vi "VNA_const_generator_spa.vi"() -> ()   [LabVIEW 2013]
panel:
  in  "?":enum32{"VNA (constant signal)"}(tab)
  in  "Power (dBm)":dbl caption="Center Freq (Hz):" min=1.0 max=19.0 format="%#.6p"
  in  "Frequency  (Hz)":dbl=20.0 caption="Center Freq (Hz):" min=1.0 max=20.0 format="%#.6p"
  in  "?":enum32{"RS generator with internal  modulation"}(tab)
  in  "Power start (dBm)":dbl=-50.0 caption="Center Freq (Hz):" min=1.0 max=20.0 format="%#.6p"
  in  "Frequency start (Hz)":dbl=2.0 caption="Center Freq (Hz):" min=1.0 max=19.0 format="%#.6p"
  in  "Power end (dBm)":dbl caption="Center Freq (Hz):" min=1.0 max=19.0 format="%#.6p"
  in  "Frequency end (Hz)":dbl=20.0 caption="Center Freq (Hz):" min=1.0 max=20.0 format="%#.6p"
  in  "power_points":i32=20 caption="Power N of points"
  in  "freq_points":i32=201 caption="Frequency N of points"
  in  "MOD frequency end  (Hz)":dbl=20.0 caption="Center Freq (Hz):" min=1.0 max=20.0 format="%#.6p"
  in  "MOD frequency start  (Hz)":dbl=20.0 caption="Center Freq (Hz):" min=1.0 max=20.0 format="%#.6p"
  in  "modulation_points":i32=20 caption="modulation N of points"
  in  "?":enum32{"SPA"}(tab)
  in  "Center freq (Hz)":dbl=-10.0 caption="Center Freq (Hz):" format="%#.6p"
  in  "Span (Hz)":dbl=-10.0 caption="Center Freq (Hz):" format="%#.6p"
  in  "RBW  (Hz)":dbl=-10.0 caption="Center Freq (Hz):" format="%#.6p"
  in  "VBW (Hz)":dbl=-10.0 caption="Center Freq (Hz):" format="%#.6p"
  in  "Points":i32=4 caption="Center Freq (Hz):"
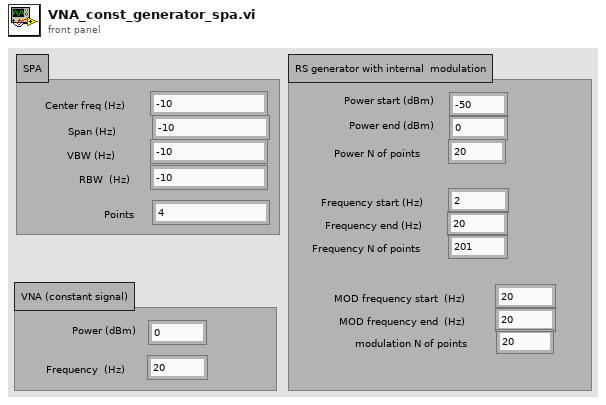
[diagram p1: front panel]
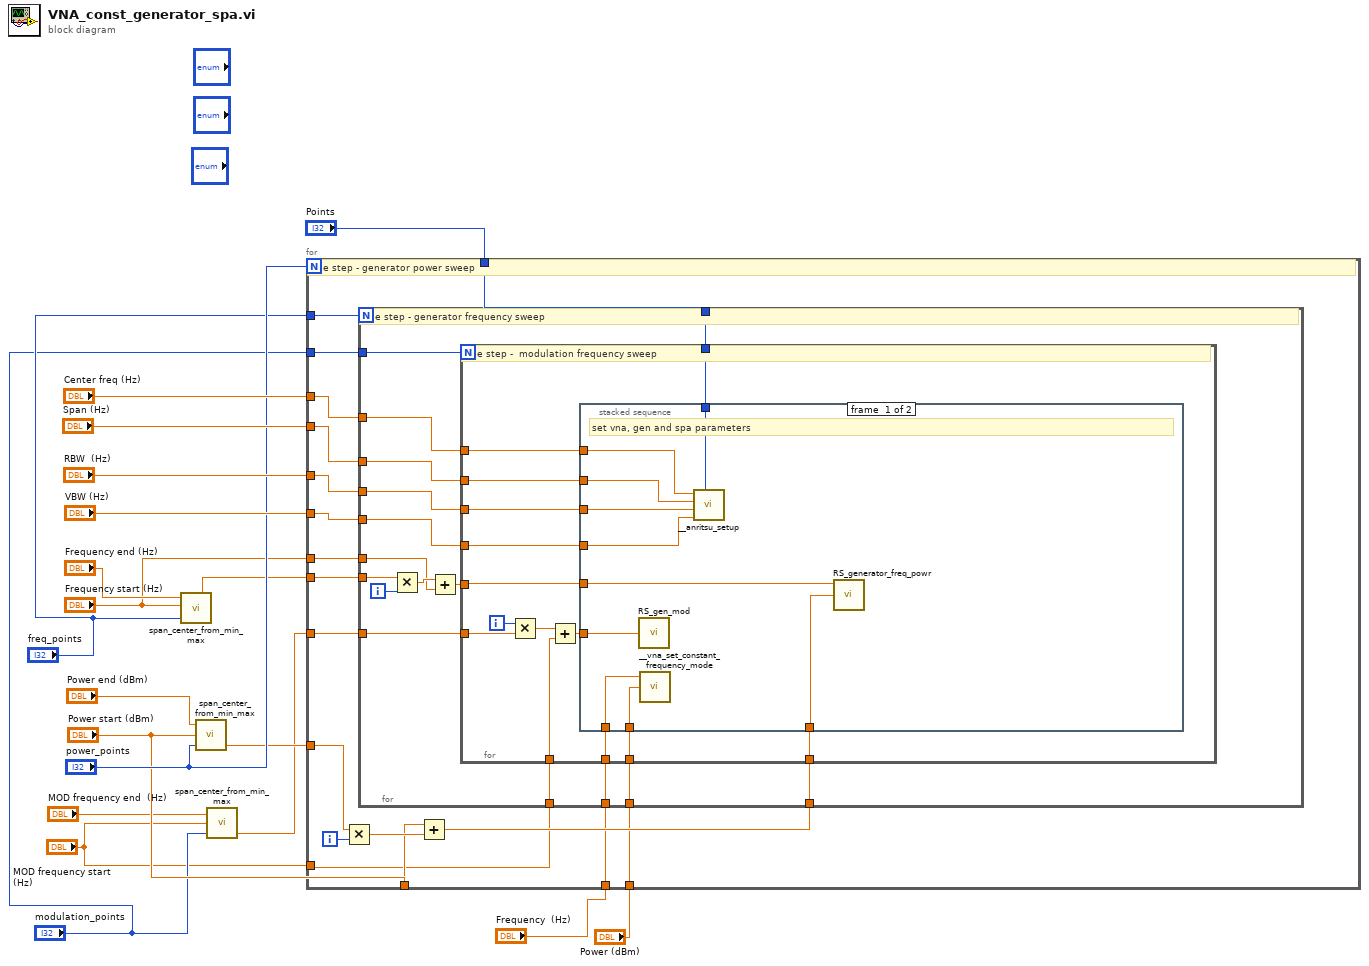
[diagram p0: block diagram]
diagram:
  n1 = call "span_center_from_min_max.vi"("No Points"="freq_points", "Begin"="Frequency start (Hz)", "End"="Frequency end (Hz)") -> ("Step"=w9:dbl)  [unwired: 2 out]
  n2 = call "span_center_from_min_max.vi"("No Points"="power_points", "Begin"="Power start (dBm)", "End"="Power end (dBm)") -> ("Step"=w12:dbl)  [unwired: 2 out]
  n3 = call "span_center_from_min_max.vi"("No Points"="modulation_points", "Begin"="MOD frequency start  (Hz)", "End"="MOD frequency end  (Hz)") -> ("Step"=w5:dbl)  [unwired: 2 out]
  n4 = for {
    N: "power_points" -> [_]
    tunnel: "Center freq (Hz)" -> [w37]
    tunnel: "Span (Hz)" -> [w36]
    tunnel: "RBW  (Hz)" -> [w35]
    tunnel: "VBW (Hz)" -> [w34]
    tunnel: "Points" -> [w33]
    tunnel: w12 -> [w30]
    tunnel: "Power start (dBm)" -> [w29]
    tunnel: w9 -> [w27]
    tunnel: "Frequency start (Hz)" -> [w26]
    tunnel: "freq_points" -> [w25]
    tunnel: w5 -> [w24]
    tunnel: "modulation_points" -> [w23]
    tunnel: "MOD frequency start  (Hz)" -> [w22]
    tunnel: "Power (dBm)" -> [w21]
    tunnel: "Frequency  (Hz)" -> [w20]
    i -> [w32]
    # "One step - generator power sweep"
    n5 = Multiply(x=w30, y=w32) -> (x*y=w31:dbl)
    n6 = Add(x=w29, y=w31) -> (x+y=w28:dbl)
    n7 = for {
      N: w25 -> [_]
      tunnel: w37 -> [w53]
      tunnel: w36 -> [w52]
      tunnel: w35 -> [w51]
      tunnel: w34 -> [w50]
      tunnel: w33 -> [w49]
      tunnel: w28 -> [w48]
      tunnel: w27 -> [w44]
      tunnel: w26 -> [w43]
      tunnel: w24 -> [w42]
      tunnel: w23 -> [w41]
      tunnel: w22 -> [w40]
      tunnel: w21 -> [w39]
      tunnel: w20 -> [w38]
      i -> [w45]
      # "One step - generator frequency sweep"
      n8 = Multiply(x=w44, y=w45) -> (x*y=w47:dbl)
      n9 = Add(x=w47, y=w43) -> (x+y=w46:dbl)
      n10 = for {
        N: w41 -> [_]
        tunnel: w53 -> [w67]
        tunnel: w52 -> [w66]
        tunnel: w51 -> [w65]
        tunnel: w50 -> [w64]
        tunnel: w49 -> [w63]
        tunnel: w48 -> [w62]
        tunnel: w46 -> [w61]
        tunnel: w42 -> [w59]
        tunnel: w40 -> [w57]
        tunnel: w39 -> [w55]
        tunnel: w38 -> [w54]
        i -> [w60]
        # "One step -  modulation frequency sweep"
        n11 = Multiply(x=w60, y=w59) -> (x*y=w58:dbl)
        n12 = Add(x=w58, y=w57) -> (x+y=w56:dbl)
        n13 = stacked-sequence {
          tunnel: w67 -> [w77 _]
          tunnel: w66 -> [w76 _]
          tunnel: w65 -> [w75 _]
          tunnel: w64 -> [w74 _]
          tunnel: w63 -> [w73 _]
          tunnel: w62 -> [w72 _]
          tunnel: w61 -> [w71 _]
          tunnel: w56 -> [w70 _]
          tunnel: w55 -> [w69 _]
          tunnel: w54 -> [w68 _]
          frame #0 {
            # "set vna, gen and spa parameters"
            n14 = call "RS_gen_mod.vi"("Internal Frequency"=w70) -> ()  [unwired: 11 in]
            n15 = call "__vna_set_constant_frequency_mode.vi"("Power dBm"=w69, "Center Freq (Hz):"=w68) -> ()  [unwired: 3 in, 1 out]
            n16 = call "__anritsu_setup.vi"("Center Freq (Hz)"=w77, "Span (Hz)"=w76, "RBW (Hz)"=w75, "VBW (Hz)"=w74, "Points"=w73) -> ()  [unwired: 1 out]
            n17 = call "RS_generator_freq_powr.vi"("Power (dBm)"=w72, "Frequnecy (Hz)"=w71) -> ()  [unwired: 1 in, 2 out]
          }
          frame #1 {
            # "show spectrum and write data to file \n                                                         show spectrum from SPA and write to file"
          }
        }
      }
    }
  }
